vi "Merge.vi"(6 "Conditional Object":refnum<class>, 8 "error in (no error)":errorcluster, 9 "Object B":refnum<class>, 10 "Object A":refnum<class>, 11 "Merge Rule in":refnum<class "Merge Rule.lvclass">) -> (0 "error out":errorcluster, 2 "Output Object":refnum<class>, 3 "Merge Rule out":refnum<class "Merge Rule.lvclass">)   [LabVIEW 2020, in "Merge Tools.lvlib" / "Merge Rule.lvclass"]
uses:
  Merge Rule.lvclass
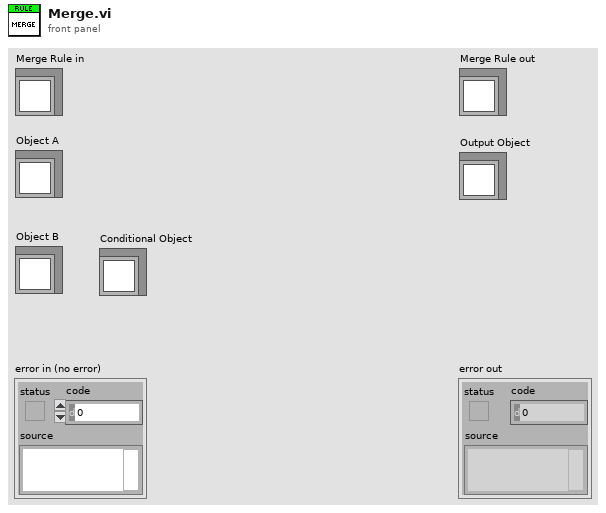
[diagram p1: front panel]
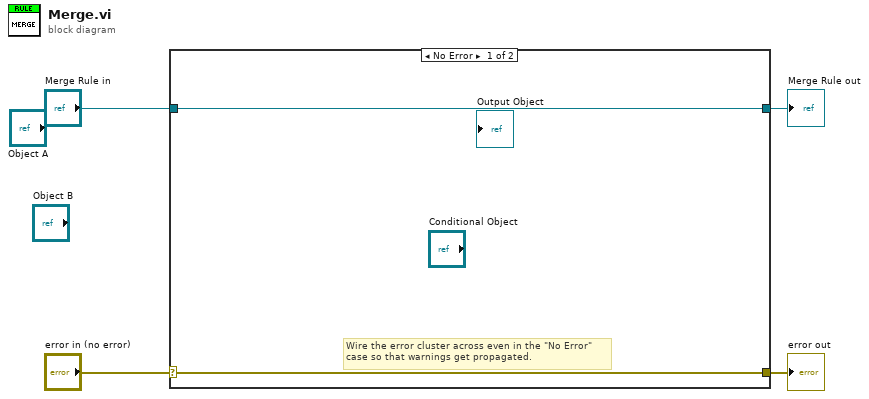
[diagram p0: block diagram]
diagram:
  n1 = case shown="No Error" "error in (no error)" {
    selector: "error in (no error)" -> [w5 w8]
    tunnel: [w5 w8] -> w3
    tunnel: [w6 w7] -> w1
    tunnel: "Merge Rule in" -> [w6 w7]
    frame No Error {
      # "Wire the error cluster across even in the \"No Error\"\ncase so that warnings get propagated."
    }
    frame Error {
    }
  }
  "error out" <- w3
  "Merge Rule out" <- w1
